vi "DelayR1_ext.vi"(6 "out":bool, 8 "T old":u32, 9 "DelayOff":u32, 10 "DelayOn":u32, 11 "R":bool) -> (0 "T old out":u32, 2 "t ms":u32, 3 "Out":bool)   [LabVIEW 2019, in "Timers.lvlib"]
uses:
  Timers.lvlib
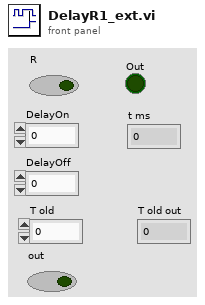
[diagram p1: front panel]
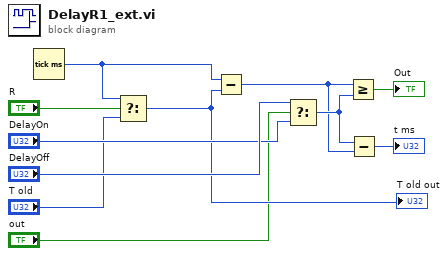
[diagram p0: block diagram]
diagram:
  n1 = Tick Count (ms)() -> (millisecond timer value=w11:u32)
  n2 = Select(t=w11, s="R", f="T old") -> (s? t:f=w3:u32)
  "T old out" <- w3
  n3 = Subtract(x=w11, y=w3) -> (x-y=w9:u32)
  n4 = Select(t="DelayOff", s="out", f="DelayOn") -> (s? t:f=w10:u32)
  n5 = Greater Or Equal?(x=w9, y=w10) -> (x >= y?=→"Out":bool)
  n6 = Subtract(x=w10, y=w9) -> (x-y=→"t ms":u32)
